vi "main.vi"   [LabVIEW 2011]
uses:
  Controls/User Event Control.ctl
  Controls/User Event Action.ctl
  Error Handling/Error Module Action.ctl
types:
  T1 = typedef "Class Objects.ctl" = cluster{"configuration":refnum<class "Configuration.lvclass">, "TDMS":refnum<class "TDMS.lvclass">[], "Power Supply":refnum<class "Power Supply.lvclass">, "Mass Flow Controller":refnum<class "Mass Flow Controller.lvclass">, "Detector":refnum<class "Detector.lvclass">}
  T2 = typedef "Error Module Action.ctl" = enum16{"Initialize", "Handle Errors", "Report Errors"}
  T3 = typedef "User Event Control.ctl" = cluster{"action":T4, "data":variant}
  T4 = typedef "User Event Action.ctl" = enum16{"Initialize", "Device Connections", "Device Settings", "Shutdown"}
  T5 = typedef "User Interface Control.ctl" = cluster{"action":T6, "data1":variant, "data2":variant}
  T6 = typedef "User Interface Action.ctl" = enum16{"Initialize", "Visibility Front Panel Controls", "Stop"}
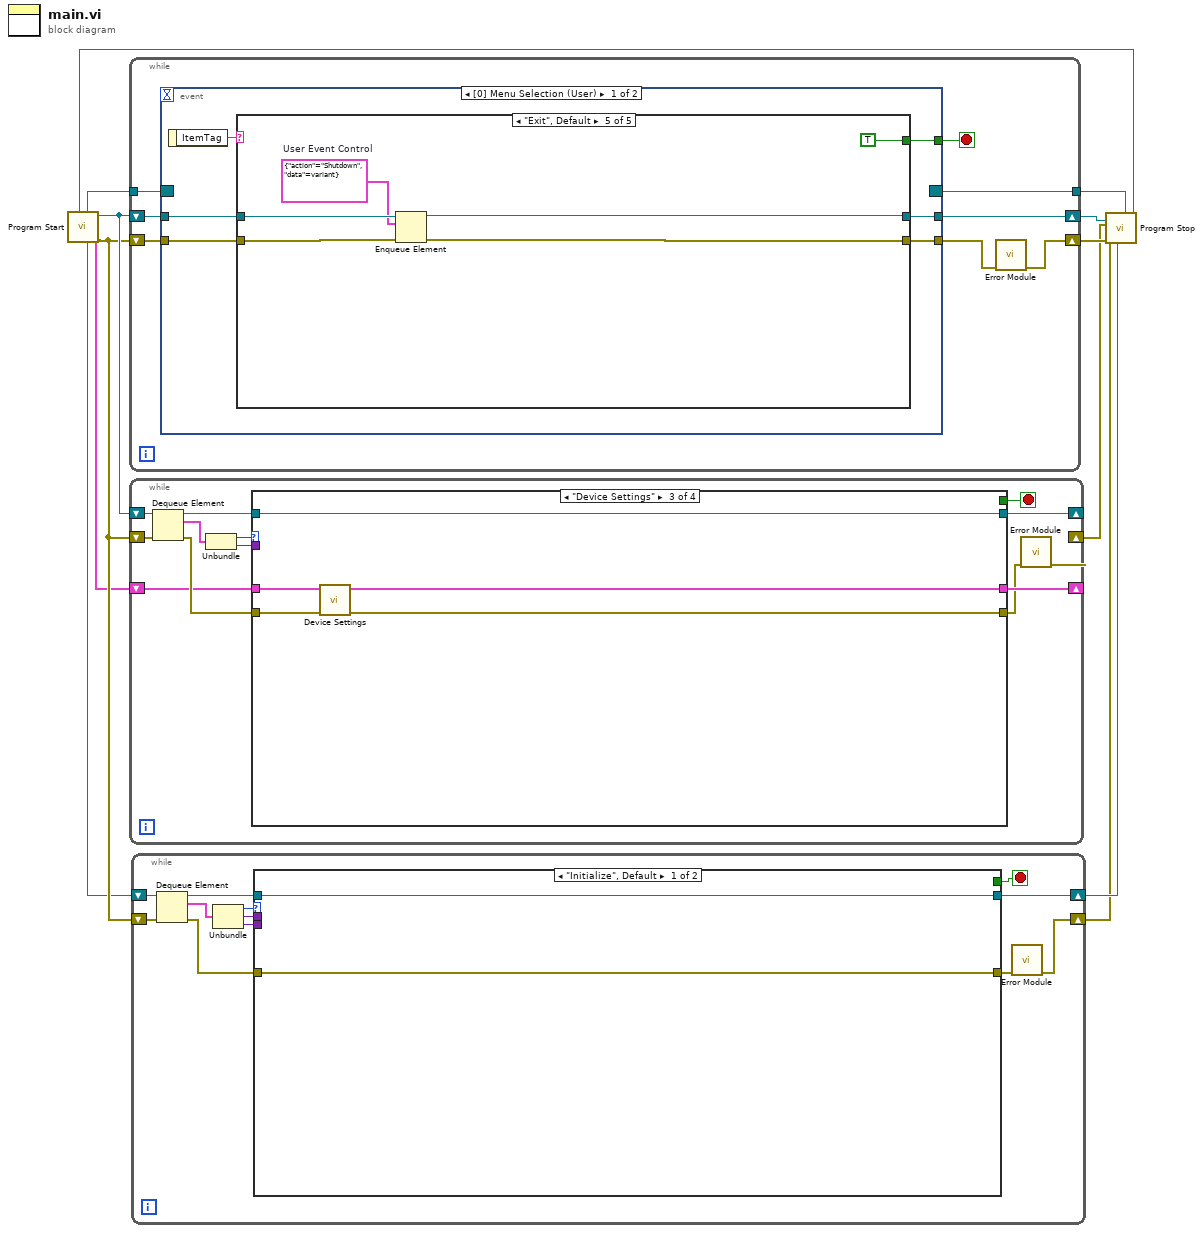
[diagram p0: block diagram]
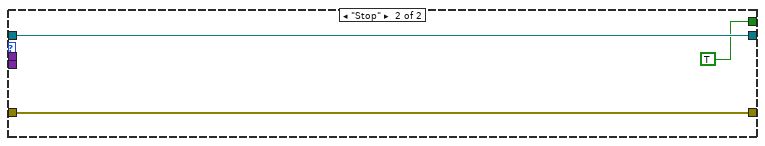
[diagram p2: hidden frame]
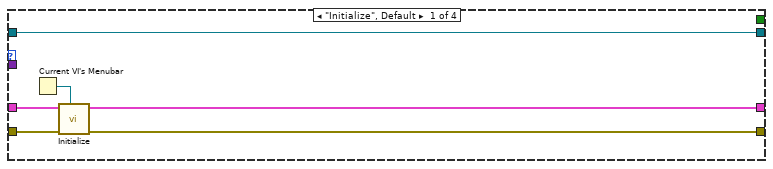
[diagram p3: hidden frame]
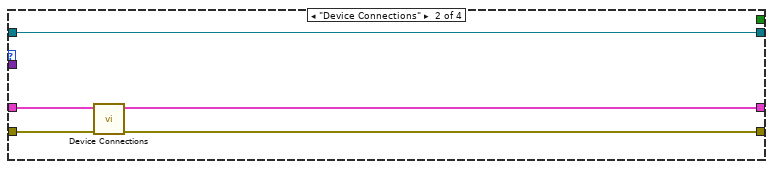
[diagram p4: hidden frame]
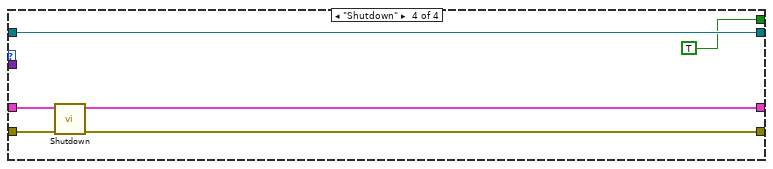
[diagram p5: hidden frame]
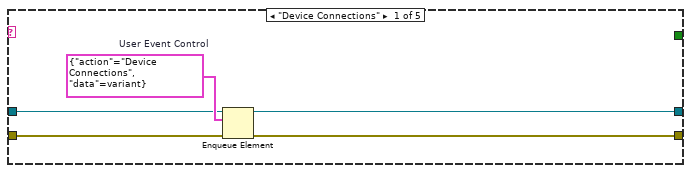
[diagram p6: hidden frame]
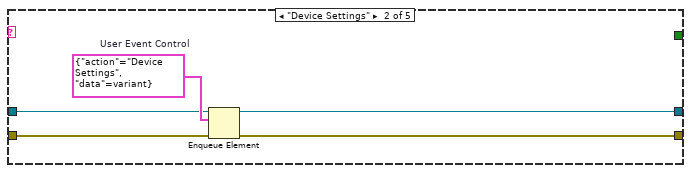
[diagram p7: hidden frame]
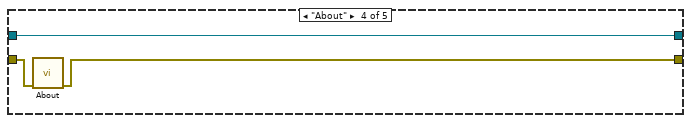
[diagram p9: hidden frame]
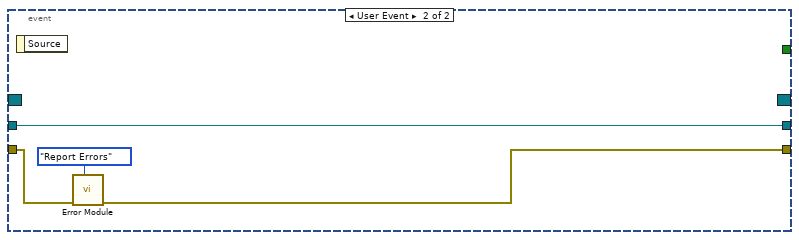
[diagram p10: hidden frame]
diagram:
  n1 = call "Program Start.vi"() -> ("error out"=w10:errorcluster, "Class Objects"=w9:T1, "user events"=w11:refnum<queue>, "user interface"=w8:refnum<queue>, "Event Registration Refnum out"=w12:refnum<event-registration>, "user event"=w6:refnum<user-event>)  [unwired: 6 in]
  n2 = while {
    tunnel: w12 -> [w20]
    tunnel: [w19] -> w5
    shift-right: [w14] -> w7
    shift-left: w11 -> [w17]
    shift-right: [w15] -> w4
    shift-left: w10 -> [w18]
    stop <- w13 stop-if-true
    n3 = event shown="[0] Menu Selection (User)" {
      selector: w20 -> [_ _]
      dyn-events: [_ _] -> w19
      timeout: _ -> [_ _]
      tunnel: w18 -> [w25 w50]
      tunnel: [w22 w48] -> w16
      tunnel: w17 -> [w24 w51]
      tunnel: [w23 w51] -> w14
      tunnel: [w21 _] -> w13
      event Menu Selection (User) {
        n4 = event-data() -> ("ItemTag"=w26:string)  [unwired: 1 in]
        n5 = case shown="\"Exit\", Default" w26 {
          tunnel: w25 -> [w29 w34 w37 w40 w47]
          tunnel: w24 -> [w30 w35 w38 w41 w46]
          tunnel: [w28 w33 w38 w41 w44] -> w23
          tunnel: [w27 w32 w37 w39 w43] -> w22
          tunnel: [_ _ _ _ TRUE] -> w21
          frame "Device Connections" {
            w31 = T3 {"action"=enum."Device Connections", "data"=variant}  # User Event Control
            n6 = Enqueue Element(queue=w30, element=w31, error in (no error)=w29) -> (queue out=w28:refnum<queue>, error out=w27:errorcluster)  [unwired: 1 in, 1 out]
          }
          frame "Device Settings" {
            w36 = T3 {"action"=enum."Device Settings", "data"=variant}  # User Event Control
            n7 = Enqueue Element(queue=w35, element=w36, error in (no error)=w34) -> (queue out=w33:refnum<queue>, error out=w32:errorcluster)  [unwired: 1 in, 1 out]
          }
          frame "Options" {
          }
          frame "About" {
            n8 = call "About.vi"("error in"=w40) -> ("error out"=w39:errorcluster)  [unwired: 10 in]
          }
          frame "Exit", Default {
            w45 = T3 {"action"=enum."Shutdown", "data"=variant}  # User Event Control
            n9 = Enqueue Element(queue=w46, element=w45, error in (no error)=w47) -> (queue out=w44:refnum<queue>, error out=w43:errorcluster)  [unwired: 1 in, 1 out]
          }
        }
      }
      event User Event {
        n10 = event-data() -> ()  [unwired: 1 in, 1 out]
        n11 = call "Error Module.vi"("Command (Handle Errors"=Error_Module_Action."Report Errors", "error in"=w50) -> ("error out"=w48:errorcluster)  [unwired: 8 in, 1 out]
      }
    }
    n12 = call "Error Module.vi"("error in"=w16) -> ("error out"=w15:errorcluster)  [unwired: 9 in, 1 out]
  }
  n13 = while {
    shift-right: [w58] -> _
    shift-left: w11 -> [w64]
    shift-right: [w56] -> w3
    shift-left: w10 -> [w63]
    shift-right: [w53] -> _
    shift-left: w9 -> [w54]
    stop <- w57 stop-if-true
    n14 = Dequeue Element(queue=w64, error in (no error)=w63) -> (queue out=w55:refnum<queue>, element=w62:T3, error out=w59:errorcluster)  [unwired: 1 in, 1 out]
    n15 = Unbundle(w62) -> ("action"=w61:T4, "data"=w60:variant)
    n16 = case shown="\"Device Settings\"" w61 {
      tunnel: w60 -> [_ _ _ _]
      tunnel: w59 -> [w70 w74 w79 w84]
      tunnel: w55 -> [w69 w71 w76 w86]
      tunnel: [w69 w71 w76 w86] -> w58
      tunnel: [w65 w72 w77 w81] -> w52
      tunnel: [_ _ _ TRUE] -> w57
      tunnel: w54 -> [w67 w75 w80 w83]
      tunnel: [w66 w73 w78 w82] -> w53
      frame "Initialize", Default {
        n17 = Current VI's Menubar() -> (w68:refnum<k9>)
        n18 = call "Initialize.vi"("menu ref"=w68, "error in"=w70, "class objects IN"=w67) -> ("error out"=w65:errorcluster, "class objects OUT"=w66:T1)  [unwired: 7 in]
      }
      frame "Device Connections" {
        n19 = call "Device Connections.vi"("error in"=w74, "objects in"=w75) -> ("error out"=w72:errorcluster, "objects out"=w73:T1)  [unwired: 8 in]
      }
      frame "Device Settings" {
        n20 = call "Device Settings.vi"("error in"=w79, "objects in"=w80) -> ("error out"=w77:errorcluster, "objects out"=w78:T1)  [unwired: 8 in]
      }
      frame "Shutdown" {
        n21 = call "Shutdown.vi"("error in"=w84, "objects in"=w83) -> ("error out"=w81:errorcluster, "objects out"=w82:T1)  [unwired: 8 in]
      }
    }
    n22 = call "Error Module.vi"("error in"=w52) -> ("error out"=w56:errorcluster)  [unwired: 9 in, 1 out]
  }
  n23 = while {
    shift-right: [w91] -> w2
    shift-left: w8 -> [w97]
    shift-right: [w88] -> w1
    shift-left: w10 -> [w98]
    stop <- w90 stop-if-true
    n24 = Dequeue Element(queue=w97, error in (no error)=w98) -> (queue out=w92:refnum<queue>, element=w96:T5, error out=w94:errorcluster)  [unwired: 1 in, 1 out]
    n25 = Unbundle(w96) -> ("action"=w95:T6, "data1"=w93:variant, "data2"=w87:variant)
    n26 = case shown="\"Initialize\", Default" w95 {
      tunnel: w94 -> [w100 w103]
      tunnel: w93 -> [_ _]
      tunnel: w92 -> [w99 w102]
      tunnel: [w99 w102] -> w91
      tunnel: [w100 w103] -> w89
      tunnel: [_ TRUE] -> w90
      tunnel: w87 -> [_ _]
      frame "Initialize", Default {
      }
      frame "Stop" {
      }
    }
    n27 = call "Error Module.vi"("error in"=w89) -> ("error out"=w88:errorcluster)  [unwired: 9 in, 1 out]
  }
  n28 = call "Program Stop.vi"("user event"=w6, "Event Registration Refnum in"=w5, "GUI queue"=w2, "control queue"=w7, "GUI error"=w1, "operation error"=w3, "control error"=w4) -> ()  [unwired: 5 in]
